vi "Accumulate waveform data.vi"(6 "max size":i32=4096, 7 "reset":bool, 8 "error in (no error)":errorcluster, 11 "data":waveform(dbl)[](array[waveform])) -> (0 "error out":errorcluster, 3 "data out":waveform(dbl)[](array[waveform]))   [LabVIEW 2013]
uses:
  <vilib>/Waveform/WDTOps.llb/WDT Append Waveforms DBL.vi
  <vilib>/Waveform/WDTOps.llb/WDT Get Waveform Subset DBL.vi
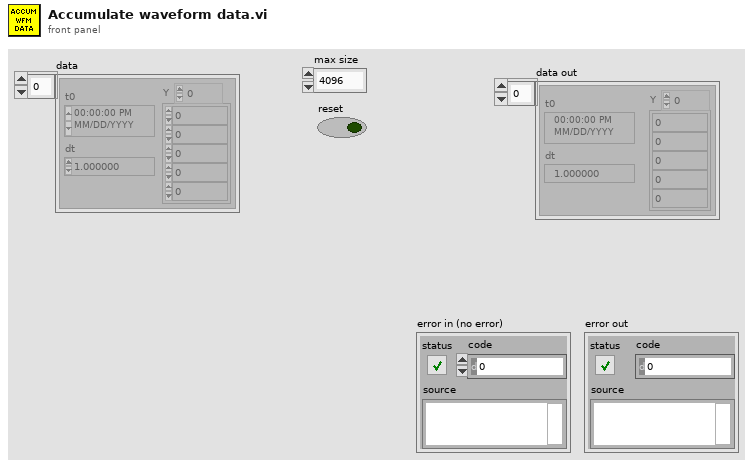
[diagram p1: front panel]
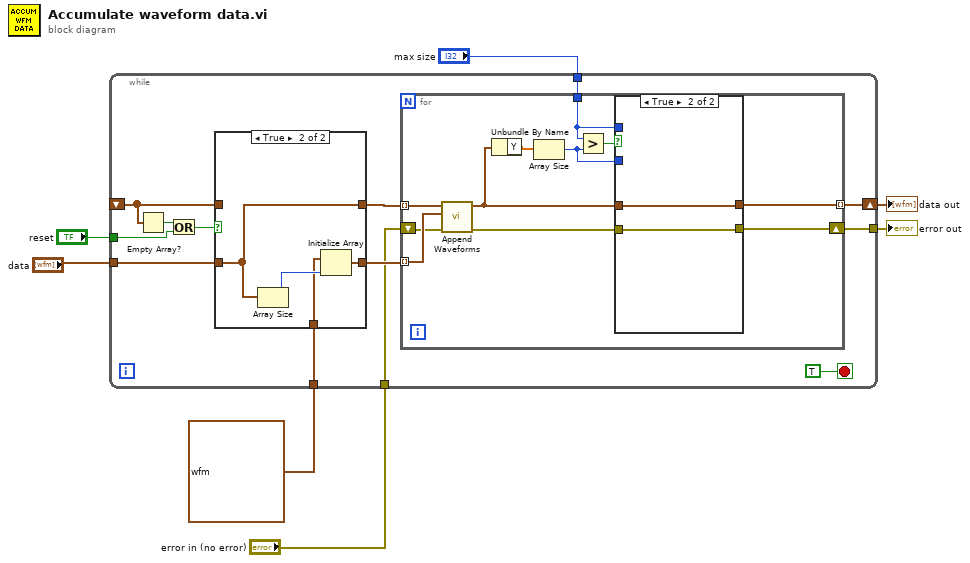
[diagram p0: block diagram]
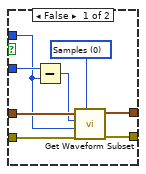
[diagram p3: hidden frame]
diagram:
  n1 = while {
    tunnel: "data" -> [w18]
    shift-right: [w20] -> w1
    shift-left: _ -> [w19]
    tunnel: "reset" -> [w13]
    tunnel: "max size" -> [w11]
    tunnel: waveform(dbl) {"t0"=timestamp(0 s since 1904-01-01), "dt"=1.0, "Y"=[]} ("motor subset") -> [w10]
    tunnel: "error in (no error)" -> [w9]
    tunnel: [w8] -> w2
    stop <- TRUE stop-if-true
    n2 = Empty Array?(array=w19) -> (empty?=w15:bool)
    n3 = Or(x=w15, y=w13) -> (x .or. y?=w14:bool)
    n4 = case shown="True" w14 {
      tunnel: w19 -> [w22 _]
      tunnel: w18 -> [w21 w26]
      tunnel: [w22 w26] -> w17
      tunnel: [w21 w24] -> w16
      tunnel: w10 -> [_ w23]
      frame False {
      }
      frame True {
        n5 = Array Size(array=w26) -> (size(s)=w25:i32)
        n6 = Initialize Array(w23, w25) -> (w24:waveform(dbl)[])
      }
    }
    n7 = for {
      tunnel: w17 -> [w34] mode=indexing
      tunnel: w16 -> [w33] mode=indexing
      tunnel: [w29] -> w20 mode=indexing
      tunnel: w11 -> [w36]
      shift-right: [w28] -> w8
      shift-left: w9 -> [w27]
      n8 = call-poly <vilib>:"Append Waveforms.vi"("error in (no error)"=w27, "waveform B"=w33, "waveform A"=w34) -> ("error out"=w30:errorcluster, "waveform out"=w31:waveform(dbl))  [unwired: 7 in]
      n9 = Unbundle By Name(w31) -> ("Y"=w32:dbl[])
      n10 = Array Size(array=w32) -> (size(s)=w35:i32)
      n11 = Greater?(x=w36, y=w35) -> (0:w37:bool)
      n12 = case shown="True" w37 {
        tunnel: w36 -> [w42 _]
        tunnel: w35 -> [w45 _]
        tunnel: w31 -> [w44 w47]
        tunnel: w30 -> [w41 w46]
        tunnel: [w39 w47] -> w29
        tunnel: [w38 w46] -> w28
        frame False {
          w40 = u16 0 items=["Samples", "Relative Time"] ("start/duration format")
          n13 = Subtract(x=w45, y=w42) -> (x-y=w43:i32)
          n14 = call-poly <vilib>:"Get Waveform Subset.vi"("start/duration format"=w40, "error in (no error)"=w41, "duration"=w42, "start samples/time"=w43, "waveform in"=w44) -> ("error out"=w38:errorcluster, "waveform out"=w39:waveform(dbl))  [unwired: 1 in, 2 out]
        }
        frame True {
        }
      }
    }
  }
  "error out" <- w2
  "data out" <- w1
